vi "comp64_test.vi"() -> ()   [LabVIEW 2016]
panel:
  out "element":u16
  out "Numeric":i32
  out "Boolean 2":bool
  in  "stop":bool
  in  "CompVal":u16 format="%x"
  in  "CompArray":u16[](array[numeric])=[2047, 2446, 2830, 3184, 3494, 3749, 3938, 4055, 4094, 4055, 3938, 3749, 3494, 3184, 2830, 2446, 2047, 1648, 1264, 910, 600, 345, 156, 39, 0, 39, 156, 345, 600, 910, 1264, 1648, 2047, 2446, 2830, 3184, 3494, 3749, 3938, 4055, 4094, 4055, 3938, 3749, 3494, 3184, 2830, 2446, 2047, 1648, 1264, 910, 600, 345, 156, 39, 0, 39, 156, 345, 600, 910, 1264, 1648]
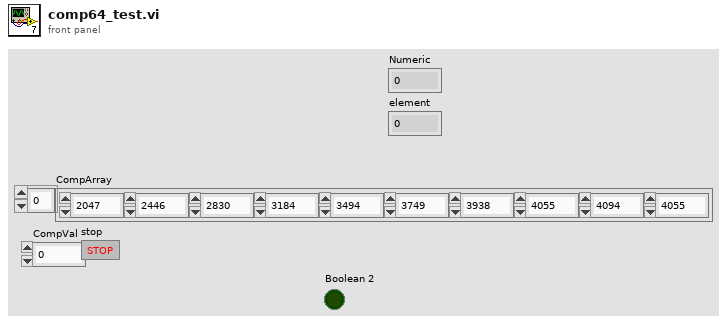
[diagram p1: front panel]
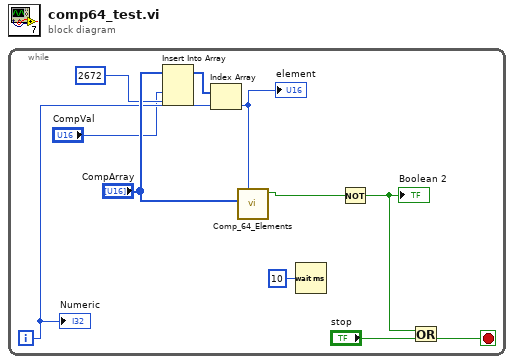
[diagram p0: block diagram]
diagram:
  n1 = while {
    i -> [w8]
    stop <- w6 stop-if-true
    n2 = Insert Into Array(array="CompArray", new element #1="CompVal", new element #2=u16 2672 ("new element/subarray")) -> (w3:u16[])  [unwired: 1 in]
    n3 = Index Array(array=w3, index=w8) -> (element=w7:u16)
    "element" <- w7
    n4 = call "Comp_64_Elements.vi"("Array"="CompArray", "CompVal"=w7) -> ("Boolean"=w5:bool)  [unwired: 9 in]
    n5 = Wait (ms)(milliseconds to wait=u32 10) -> ()  [unwired: 1 out]
    n6 = Not(x=w5) -> (.not. x?=w4:bool)
    "Boolean 2" <- w4
    n7 = Or(x=w4, y="stop") -> (x .or. y?=w6:bool)
    "Numeric" <- w8
  }
